vi "Multi1Darray.vi"() -> ()   [LabVIEW 2014]
uses:
  <vilib>/Analysis/baseanly.llb/Mean (DBL).vi
  <vilib>/Utility/file.llb/Read From Spreadsheet File (DBL).vi
  <vilib>/Analysis/NI_AALBase.lvlib
panel:
  out "Array":dbl[][](array[numeric])
  in  "Frame-rate correction":bool
  out "output array":path[][](array[path])=[[path "E:/MALDI Plots/02_14_24_data_18_spot_5_DHB_electrons_dwellandSample_5000_mcp_1850_phosphor_5500_range_2V_lens1_500_pump1.2probe0.2_4ps_3to48_backward_VelAcc_1_202402141810Cameracounts.dat"], [path "E:/MALDI Plots/02_14_24_data_14_spot_5_DHB_electrons_dwellandSample_5000_mcp_1850_phosphor_5500_range_2V_lens1_500_pump1.0probe0.2_4ps_3to48_backward_VelAcc_1_202402141718Cameracounts.dat"], [path "E:/MALDI Plots/02_14_24_data_12_spot_5_DHB_electrons_dwellandSample_5000_mcp_1850_phosphor_5500_range_2V_lens1_500_pump0.8probe0.2_4ps_3to48_backward_VelAcc_1_202402141651Cameracounts.dat"], [path "E:/MALDI Plots/02_14_24_data_10_spot_5_DHB_electrons_dwellandSample_5000_mcp_1850_phosphor_5500_range_2V_lens1_500_pump0.6probe0.2_4ps_3to48_backward_VelAcc_1_202402141629Cameracounts.dat"], [path "E:/MALDI Plots/02_14_24_data_2_spot_5_DHB_electrons_dwellandSample_5000_mcp_1850_phosphor_5500_range_2V_lens1_500_pump0.4probe0.2_4ps_3to48_backward_VelAcc_1_202402141222Cameracounts.dat"], [path "E:/MALDI Plots/02_13_24_data_6_spot_3_DHB_electrons_dwellandSample_5000_mcp_1850_phosphor_5500_range_2V_lens1_500_pump0.2probe0.2_1by1_4ps_3to48_backward_VelAcc_1_202402131406Cameracounts.dat"], [path ""], [path ""], [path ""]]
  in  "Stop Button":bool
  in  "start path":path=path "E:/MALDI Plots"
  in  "Tab Control":T1(tab)=enum."Combine Graph of 9 Plots"
  out "Waveform Graph 0":dbl[](graph)=[1.257, 1.248, 1.265, 1.215, 1.222, 1.21, 1.235, 1.2, 1.224, 1.247, 1.211, 1.189, 1.237, 1.208, 1.206, 1.211, 1.179, 1.203, 1.224, 1.217, 1.188, 1.224, 1.277, 1.3, 1.324, 1.333, 1.284, 1.238, 1.221, 1.215, 1.246, 1.229, 1.209, 1.228, 1.221, 1.194, 1.166, 1.215, 1.214, 1.184, 1.186, 1.221, 1.226, 1.218, 1.208, 1.187, 1.209, 1.166, 1.151, 1.201, 1.185, 1.164, 1.17, 1.155, 1.165, 1.181, 1.154, 1.211, 1.189, 1.174, 1.171, 1.169, 1.125, 1.173, 1.152, 1.2, 1.186, 1.178, 1.17, 1.166, 1.177, 1.171, 1.15, 1.15, 1.18]
  out "Waveform Graph 1":dbl[](graph)=[1.046, 1.067, 1.047, 1.058, 1.069, 1.074, 1.062, 1.069, 1.082, 1.057, 1.067, 1.081, 1.074, 1.099, 1.054, 1.069, 1.086, 1.073, 1.083, 1.068, 1.074, 1.106, 1.161, 1.261, 1.324, 1.33, 1.285, 1.249, 1.192, 1.194, 1.201, 1.196, 1.166, 1.155, 1.157, 1.152, 1.168, 1.131, 1.138, 1.109, 1.122, 1.112, 1.124, 1.086, 1.117, 1.102, 1.09, 1.096, 1.095, 1.098, 1.041, 1.053, 1.054, 1.061, 1.056, 1.057, 1.084, 1.074, 1.063, 1.061, 1.053, 1.052, 1.039, 1.042, 1.068, 1.058, 1.08, 1.082, 1.023, 1.028, 1.021, 1.008, 1.005, 1.05, 1.041]
  out "Waveform Graph 3":dbl[](graph)=[0.779, 0.736, 0.746, 0.749, 0.715, 0.75, 0.745, 0.769, 0.746, 0.78, 0.767, 0.765, 0.753, 0.755, 0.768, 0.746, 0.76, 0.76, 0.785, 0.784, 0.788, 0.772, 0.855, 0.958, 1.047, 1.097, 1.057, 1.034, 0.981, 0.982, 0.972, 0.963, 0.928, 0.922, 0.92, 0.915, 0.926, 0.887, 0.886, 0.869, 0.84, 0.84, 0.832, 0.822, 0.827, 0.816, 0.815, 0.831, 0.809, 0.816, 0.817, 0.805, 0.774, 0.765, 0.793, 0.83, 0.824, 0.802, 0.759, 0.776, 0.764, 0.743, 0.775, 0.762, 0.76, 0.77, 0.784, 0.761, 0.777, 0.763, 0.739, 0.746, 0.766, 0.746, 0.741]
  out "Waveform Graph 4":dbl[](graph)=[0.59, 0.604, 0.602, 0.59, 0.576, 0.579, 0.57, 0.581, 0.568, 0.579, 0.543, 0.58, 0.591, 0.577, 0.582, 0.563, 0.584, 0.591, 0.564, 0.571, 0.591, 0.625, 0.674, 0.786, 0.91, 0.973, 0.964, 0.935, 0.917, 0.899, 0.874, 0.844, 0.852, 0.817, 0.818, 0.8, 0.796, 0.769, 0.748, 0.732, 0.724, 0.717, 0.73, 0.699, 0.708, 0.685, 0.696, 0.701, 0.689, 0.651, 0.655, 0.663, 0.64, 0.653, 0.648, 0.665, 0.661, 0.616, 0.623, 0.634, 0.621, 0.633, 0.622, 0.617, 0.624, 0.614, 0.593, 0.606, 0.604, 0.573, 0.604, 0.586, 0.58, 0.558, 0.588]
  out "Waveform Graph 5":dbl[](graph)=[0.44, 0.48, 0.463, 0.455, 0.461, 0.469, 0.475, 0.477, 0.479, 0.482, 0.481, 0.477, 0.492, 0.492, 0.497, 0.495, 0.497, 0.511, 0.51, 0.503, 0.528, 0.535, 0.606, 0.734, 0.892, 0.981, 1.019, 0.964, 0.934, 0.887, 0.862, 0.851, 0.824, 0.85, 0.818, 0.791, 0.821, 0.761, 0.744, 0.739, 0.736, 0.722, 0.742, 0.681, 0.685, 0.668, 0.664, 0.678, 0.661, 0.643, 0.64, 0.644, 0.629, 0.601, 0.605, 0.594, 0.621, 0.612, 0.58, 0.546, 0.578, 0.569, 0.564, 0.58, 0.593, 0.569, 0.566, 0.559, 0.554, 0.555, 0.527, 0.518, 0.541, 0.541, 0.519]
  out "Waveform Graph 2":dbl[](graph)=[0.941, 0.927, 0.925, 0.947, 0.959, 0.926, 0.936, 0.927, 0.92, 0.909, 0.917, 0.929, 0.929, 0.912, 0.92, 0.92, 0.962, 0.937, 0.954, 0.958, 0.964, 0.964, 1.026, 1.13, 1.212, 1.247, 1.191, 1.156, 1.153, 1.094, 1.101, 1.071, 1.06, 1.046, 1.065, 1.035, 1.034, 1.025, 1.017, 1.015, 0.989, 1.009, 0.982, 0.977, 0.961, 0.994, 0.968, 0.948, 0.963, 0.964, 0.983, 0.924, 0.957, 0.947, 0.926, 0.94, 0.915, 0.942, 0.931, 0.916, 0.915, 0.922, 0.944, 0.907, 0.943, 0.922, 0.924, 0.916, 0.917, 0.919, 0.91, 0.911, 0.907, 0.9, 0.898]
  out "Waveform Graph 6":dbl[](graph)
  out "Waveform Graph 7":dbl[](graph)
  out "Waveform Graph 8":dbl[](graph)
  in  "Normalization method":u16(ring) items=["Raw Data", "Normalize to the peak", "Normalize to the baseline"]
  out "?":dbl[][](graph)=[[1.257, 1.248, 1.265, 1.215, 1.222, 1.21, 1.235, 1.2, 1.224, 1.247, 1.211, 1.189, 1.237, 1.208, 1.206, 1.211, 1.179, 1.203, 1.224, 1.217, 1.188, 1.224, 1.277, 1.3, 1.324, 1.333, 1.284, 1.238, 1.221, 1.215, 1.246, 1.229, 1.209, 1.228, 1.221, 1.194, 1.166, 1.215, 1.214, 1.184, 1.186, 1.221, 1.226, 1.218, 1.208, 1.187, 1.209, 1.166, 1.151, 1.201, 1.185, 1.164, 1.17, 1.155, 1.165, 1.181, 1.154, 1.211, 1.189, 1.174, 1.171, 1.169, 1.125, 1.173, 1.152, 1.2, 1.186, 1.178, 1.17, 1.166, 1.177, 1.171, 1.15, 1.15, 1.18], [1.046, 1.067, 1.047, 1.058, 1.069, 1.074, 1.062, 1.069, 1.082, 1.057, 1.067, 1.081, 1.074, 1.099, 1.054, 1.069, 1.086, 1.073, 1.083, 1.068, 1.074, 1.106, 1.161, 1.261, 1.324, 1.33, 1.285, 1.249, 1.192, 1.194, 1.201, 1.196, 1.166, 1.155, 1.157, 1.152, 1.168, 1.131, 1.138, 1.109, 1.122, 1.112, 1.124, 1.086, 1.117, 1.102, 1.09, 1.096, 1.095, 1.098, 1.041, 1.053, 1.054, 1.061, 1.056, 1.057, 1.084, 1.074, 1.063, 1.061, 1.053, 1.052, 1.039, 1.042, 1.068, 1.058, 1.08, 1.082, 1.023, 1.028, 1.021, 1.008, 1.005, 1.05, 1.041], [0.941, 0.927, 0.925, 0.947, 0.959, 0.926, 0.936, 0.927, 0.92, 0.909, 0.917, 0.929, 0.929, 0.912, 0.92, 0.92, 0.962, 0.937, 0.954, 0.958, 0.964, 0.964, 1.026, 1.13, 1.212, 1.247, 1.191, 1.156, 1.153, 1.094, 1.101, 1.071, 1.06, 1.046, 1.065, 1.035, 1.034, 1.025, 1.017, 1.015, 0.989, 1.009, 0.982, 0.977, 0.961, 0.994, 0.968, 0.948, 0.963, 0.964, 0.983, 0.924, 0.957, 0.947, 0.926, 0.94, 0.915, 0.942, 0.931, 0.916, 0.915, 0.922, 0.944, 0.907, 0.943, 0.922, 0.924, 0.916, 0.917, 0.919, 0.91, 0.911, 0.907, 0.9, 0.898], [0.779, 0.736, 0.746, 0.749, 0.715, 0.75, 0.745, 0.769, 0.746, 0.78, 0.767, 0.765, 0.753, 0.755, 0.768, 0.746, 0.76, 0.76, 0.785, 0.784, 0.788, 0.772, 0.855, 0.958, 1.047, 1.097, 1.057, 1.034, 0.981, 0.982, 0.972, 0.963, 0.928, 0.922, 0.92, 0.915, 0.926, 0.887, 0.886, 0.869, 0.84, 0.84, 0.832, 0.822, 0.827, 0.816, 0.815, 0.831, 0.809, 0.816, 0.817, 0.805, 0.774, 0.765, 0.793, 0.83, 0.824, 0.802, 0.759, 0.776, 0.764, 0.743, 0.775, 0.762, 0.76, 0.77, 0.784, 0.761, 0.777, 0.763, 0.739, 0.746, 0.766, 0.746, 0.741], [0.59, 0.604, 0.602, 0.59, 0.576, 0.579, 0.57, 0.581, 0.568, 0.579, 0.543, 0.58, 0.591, 0.577, 0.582, 0.563, 0.584, 0.591, 0.564, 0.571, 0.591, 0.625, 0.674, 0.786, 0.91, 0.973, 0.964, 0.935, 0.917, 0.899, 0.874, 0.844, 0.852, 0.817, 0.818, 0.8, 0.796, 0.769, 0.748, 0.732, 0.724, 0.717, 0.73, 0.699, 0.708, 0.685, 0.696, 0.701, 0.689, 0.651, 0.655, 0.663, 0.64, 0.653, 0.648, 0.665, 0.661, 0.616, 0.623, 0.634, 0.621, 0.633, 0.622, 0.617, 0.624, 0.614, 0.593, 0.606, 0.604, 0.573, 0.604, 0.586, 0.58, 0.558, 0.588], [0.44, 0.48, 0.463, 0.455, 0.461, 0.469, 0.475, 0.477, 0.479, 0.482, 0.481, 0.477, 0.492, 0.492, 0.497, 0.495, 0.497, 0.511, 0.51, 0.503, 0.528, 0.535, 0.606, 0.734, 0.892, 0.981, 1.019, 0.964, 0.934, 0.887, 0.862, 0.851, 0.824, 0.85, 0.818, 0.791, 0.821, 0.761, 0.744, 0.739, 0.736, 0.722, 0.742, 0.681, 0.685, 0.668, 0.664, 0.678, 0.661, 0.643, 0.64, 0.644, 0.629, 0.601, 0.605, 0.594, 0.621, 0.612, 0.58, 0.546, 0.578, 0.569, 0.564, 0.58, 0.593, 0.569, 0.566, 0.559, 0.554, 0.555, 0.527, 0.518, 0.541, 0.541, 0.519]]
  in  "Index":dbl
  in  "Length":dbl=150.0
  in  "Plot 1":u16(ring) items=["Plot 0", "Plot 1", "Plot 2", "Plot 3", "Plot 4", "Plot 5", "Plot 6", "Plot 7", "Plot 8"]
  in  "Feature On/Off":bool
  out "Combine graph 1":dbl[][](graph)=[[0.642, 0.631, 0.634, 0.632, 0.656, 0.666, 0.681, 0.659, 0.655, 0.66, 0.654, 0.682, 0.672, 0.695, 0.687, 0.674, 0.684, 0.688, 0.68, 0.693, 0.713, 0.731, 0.838, 1.072, 1.319, 1.442, 1.33, 1.313, 1.262, 1.224, 1.197, 1.191, 1.155, 1.137, 1.115, 1.122, 1.103, 1.1, 1.065, 1.058, 1.053, 1.007, 0.99, 0.942, 0.964, 0.979, 0.983, 0.953, 0.955, 0.977, 0.915, 0.931, 0.907, 0.912, 0.893, 0.91, 0.896, 0.927, 0.855, 0.878, 0.851, 0.854, 0.851, 0.839, 0.875, 0.828, 0.83, 0.804, 0.839, 0.834, 0.815, 0.791, 0.784, 0.784, 0.784], [0.634318732525629, 0.6625405405405406, 0.6517893755824791, 0.6168480894687792, 0.6585088536812675, 0.6611966449207829, 0.6625405405405406, 0.6571649580615098, 0.6544771668219944, 0.6719478098788444, 0.6706039142590866, 0.6732917054986021, 0.6638844361602982, 0.630287045666356, 0.6638844361602982, 0.6450698974836906, 0.6558210624417521, 0.6719478098788444, 0.6638844361602982, 0.6504454799627213, 0.6638844361602982, 0.6370065237651444, 0.6289431500465984, 0.7176402609506058, 0.936695246971109, 1.1624697110904008, 1.3559906803355077, 1.4057148182665424, 1.442, 1.3707735321528425, 1.394963653308481, 1.321049394221808, 1.358678471575023, 1.3237371854613234, 1.307610438024231, 1.278044734389562, 1.2740130475302889, 1.268637465051258, 1.2807325256290774, 1.186659832246039, 1.235040074557316, 1.2054743709226468, 1.1449990680335507, 1.153062441752097, 1.1369356943150046, 1.1221528424976701, 1.1033383038210625, 1.0898993476234857, 1.1019944082013047, 1.0952749301025164, 1.0858676607642126, 1.067053122087605, 1.0482385834109973, 1.0253923578751165, 0.9796999068033551, 0.9891071761416589, 1.0038900279589935, 0.9917949673811742, 0.9891071761416589, 0.9917949673811742, 0.9810438024231127, 0.9501342031686859, 0.9487903075489281, 0.9595414725069897, 0.9689487418452936, 0.9581975768872321, 0.9635731593662628, 0.9783560111835973, 0.9985144454799627, 0.9770121155638397, 0.9877632805219012, 0.9783560111835973, 0.9837315936626282, 0.9985144454799627, 1.0065778191985089]]
  in  "Offset":i32
  in  "Reverse":bool=TRUE
  in  "Select the plots to average":u16(ring)=2 items=["Plot 0", "Plot 1", "Plot 0 and Plot 1"]
  in  "Average criteria":i32=1
  in  "Plot 2":u16(ring) items=["Plot 0", "Plot 1", "Plot 2", "Plot 3", "Plot 4", "Plot 5", "Plot 6", "Plot 7", "Plot 8"]
  in  "Feature On/Off":bool
  out "Waveform Graph 10":dbl[][](graph)
  in  "Array 2":dbl[](array[numeric])
  in  "Length":dbl
  in  "Index":dbl
  out "best fit parameters":dbl[](array[numeric])
  out "Decay time constant from d":dbl=inf
  out "Decay time constant from b":dbl=inf
  out "XY Graph":cluster{dbl[], dbl[]}[](graph)
  in  "Step size (us)":dbl
  in  "Initial delay (us)":dbl
  # "Plot 0"
  # "Plot 1"
  # "Plot 2"
  # "Plot 3"
  # "Plot 4"
  # "Plot 5"
  # "Plot 6"
  # "Plot 7"
  # "Plot 8"
  # "a"
  # "b"
  # "c"
  # "d"
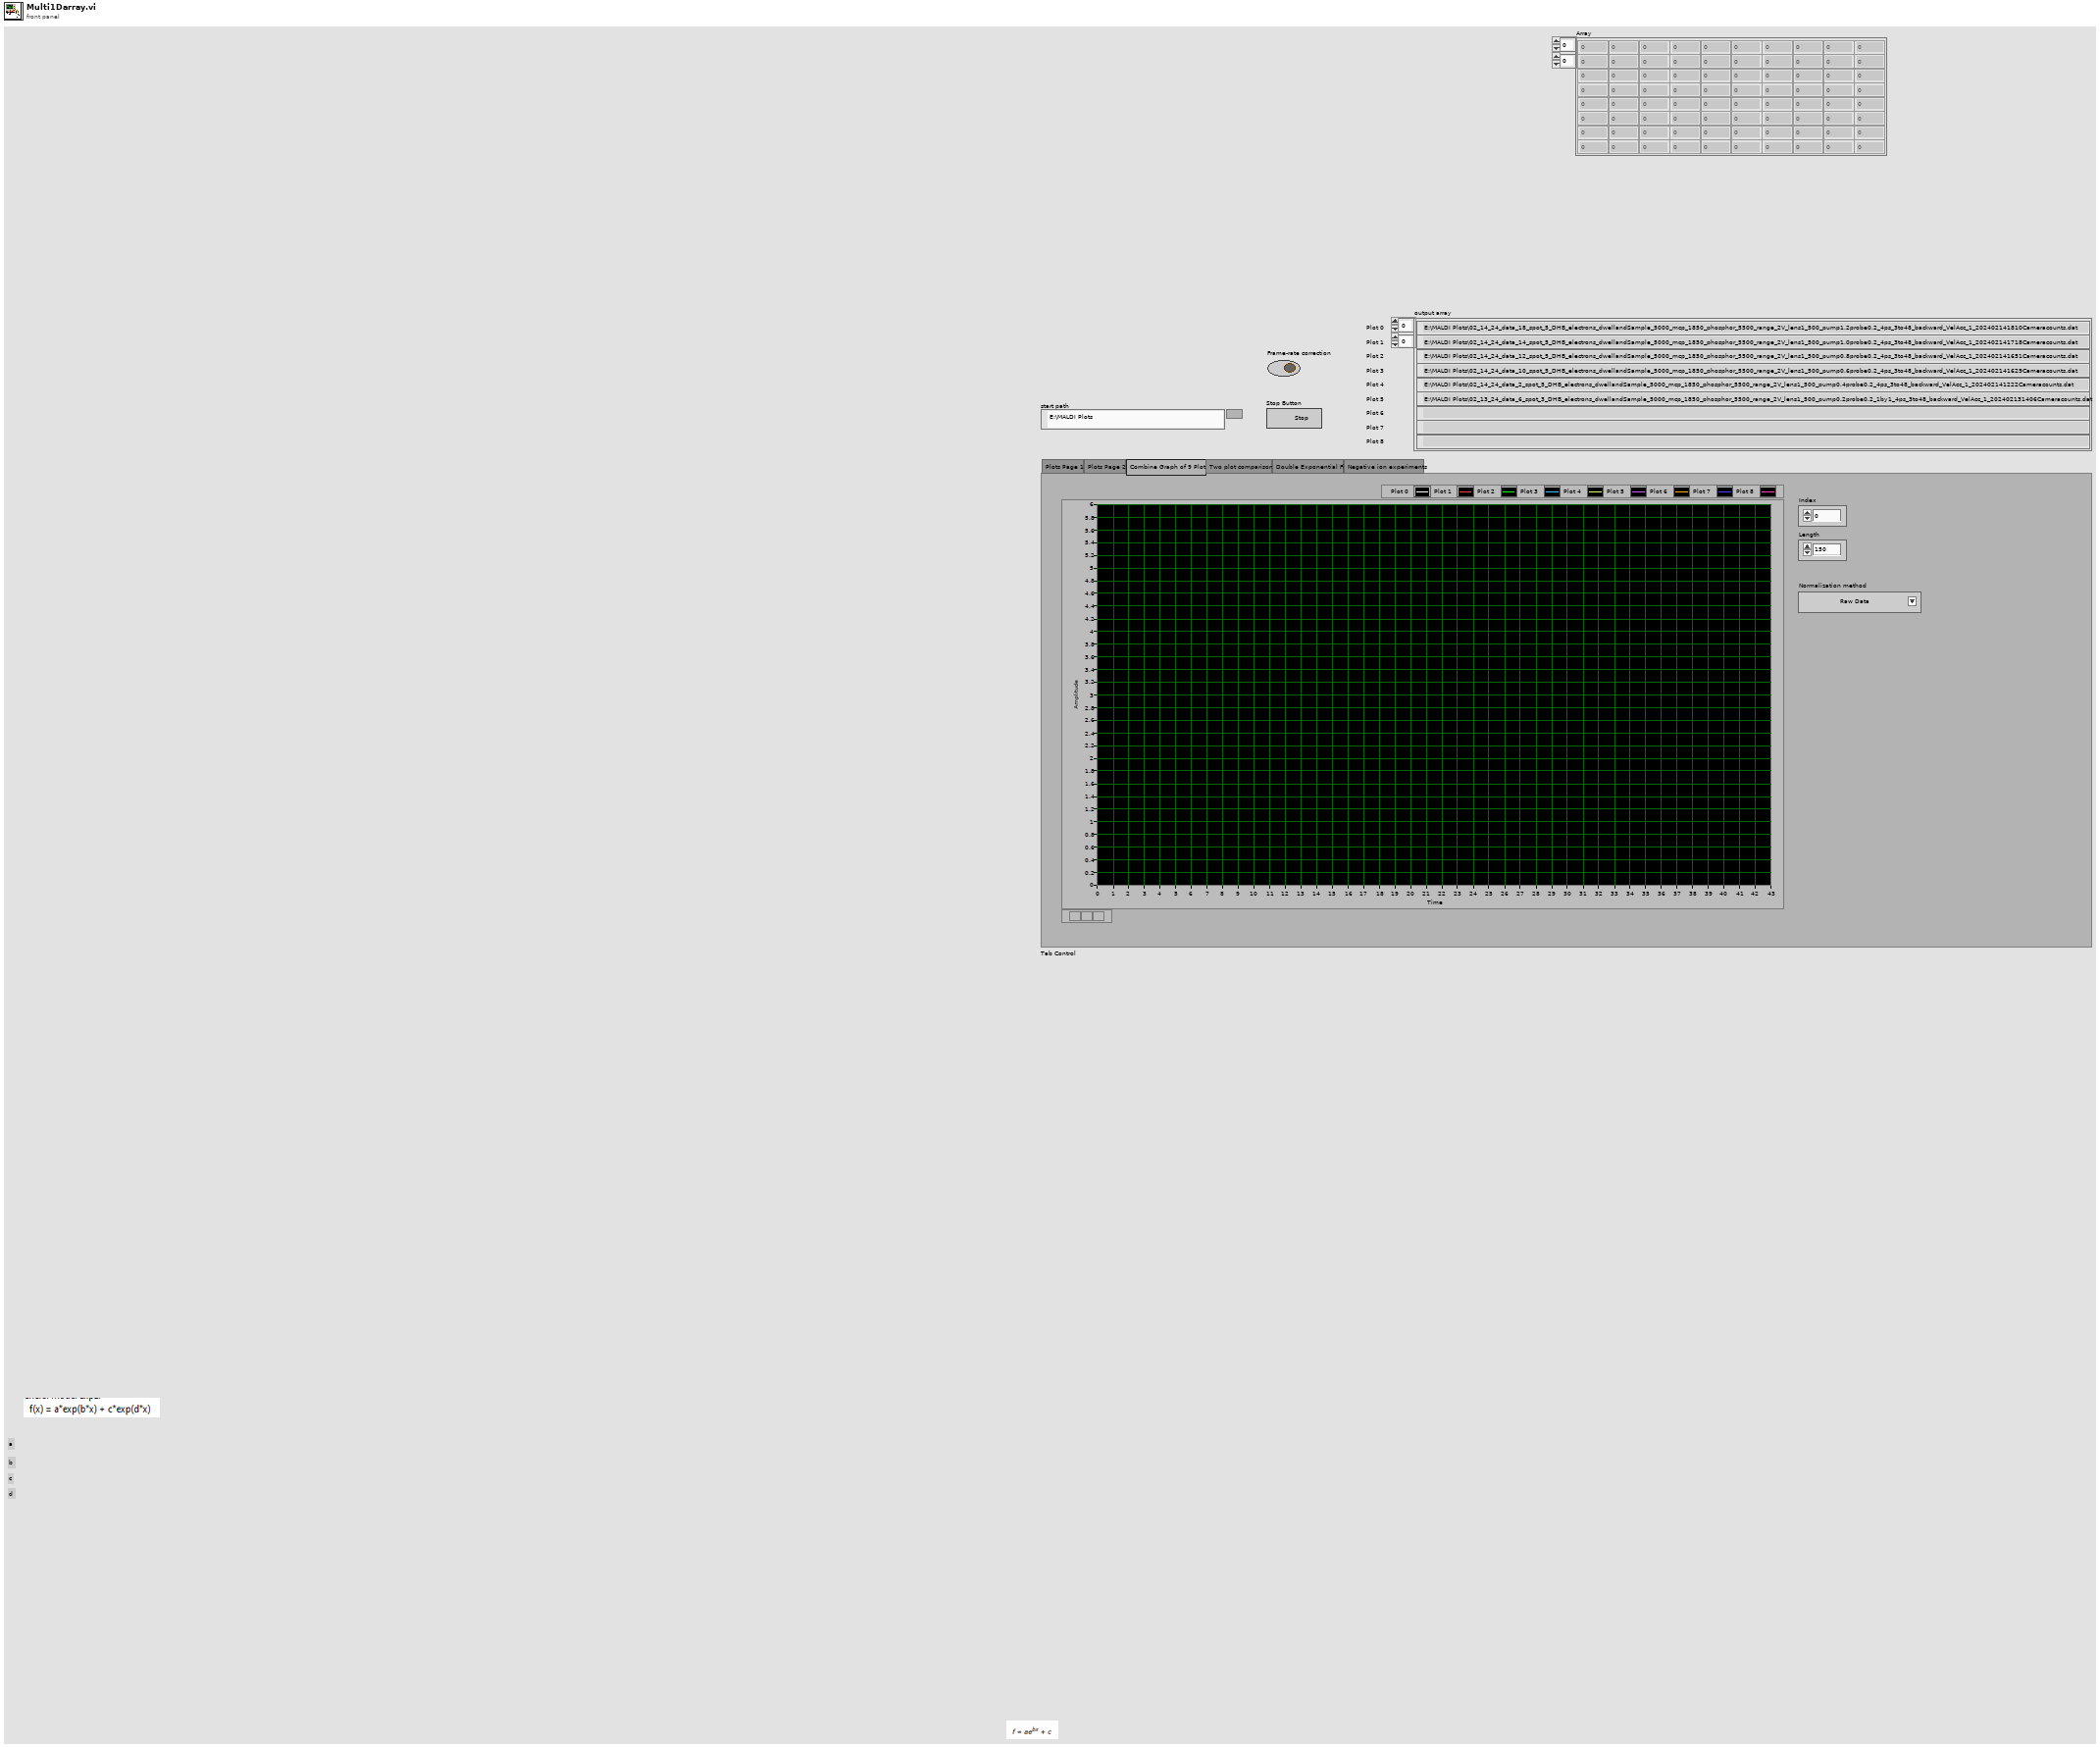
[diagram p1: front panel]
types:
  T1 = enum32{"Plots Page 1", "Plots Page 2", "Combine Graph of 9 Plots", "Two plot comparison", "Double Exponential Fit", "Negative ion experiments"}
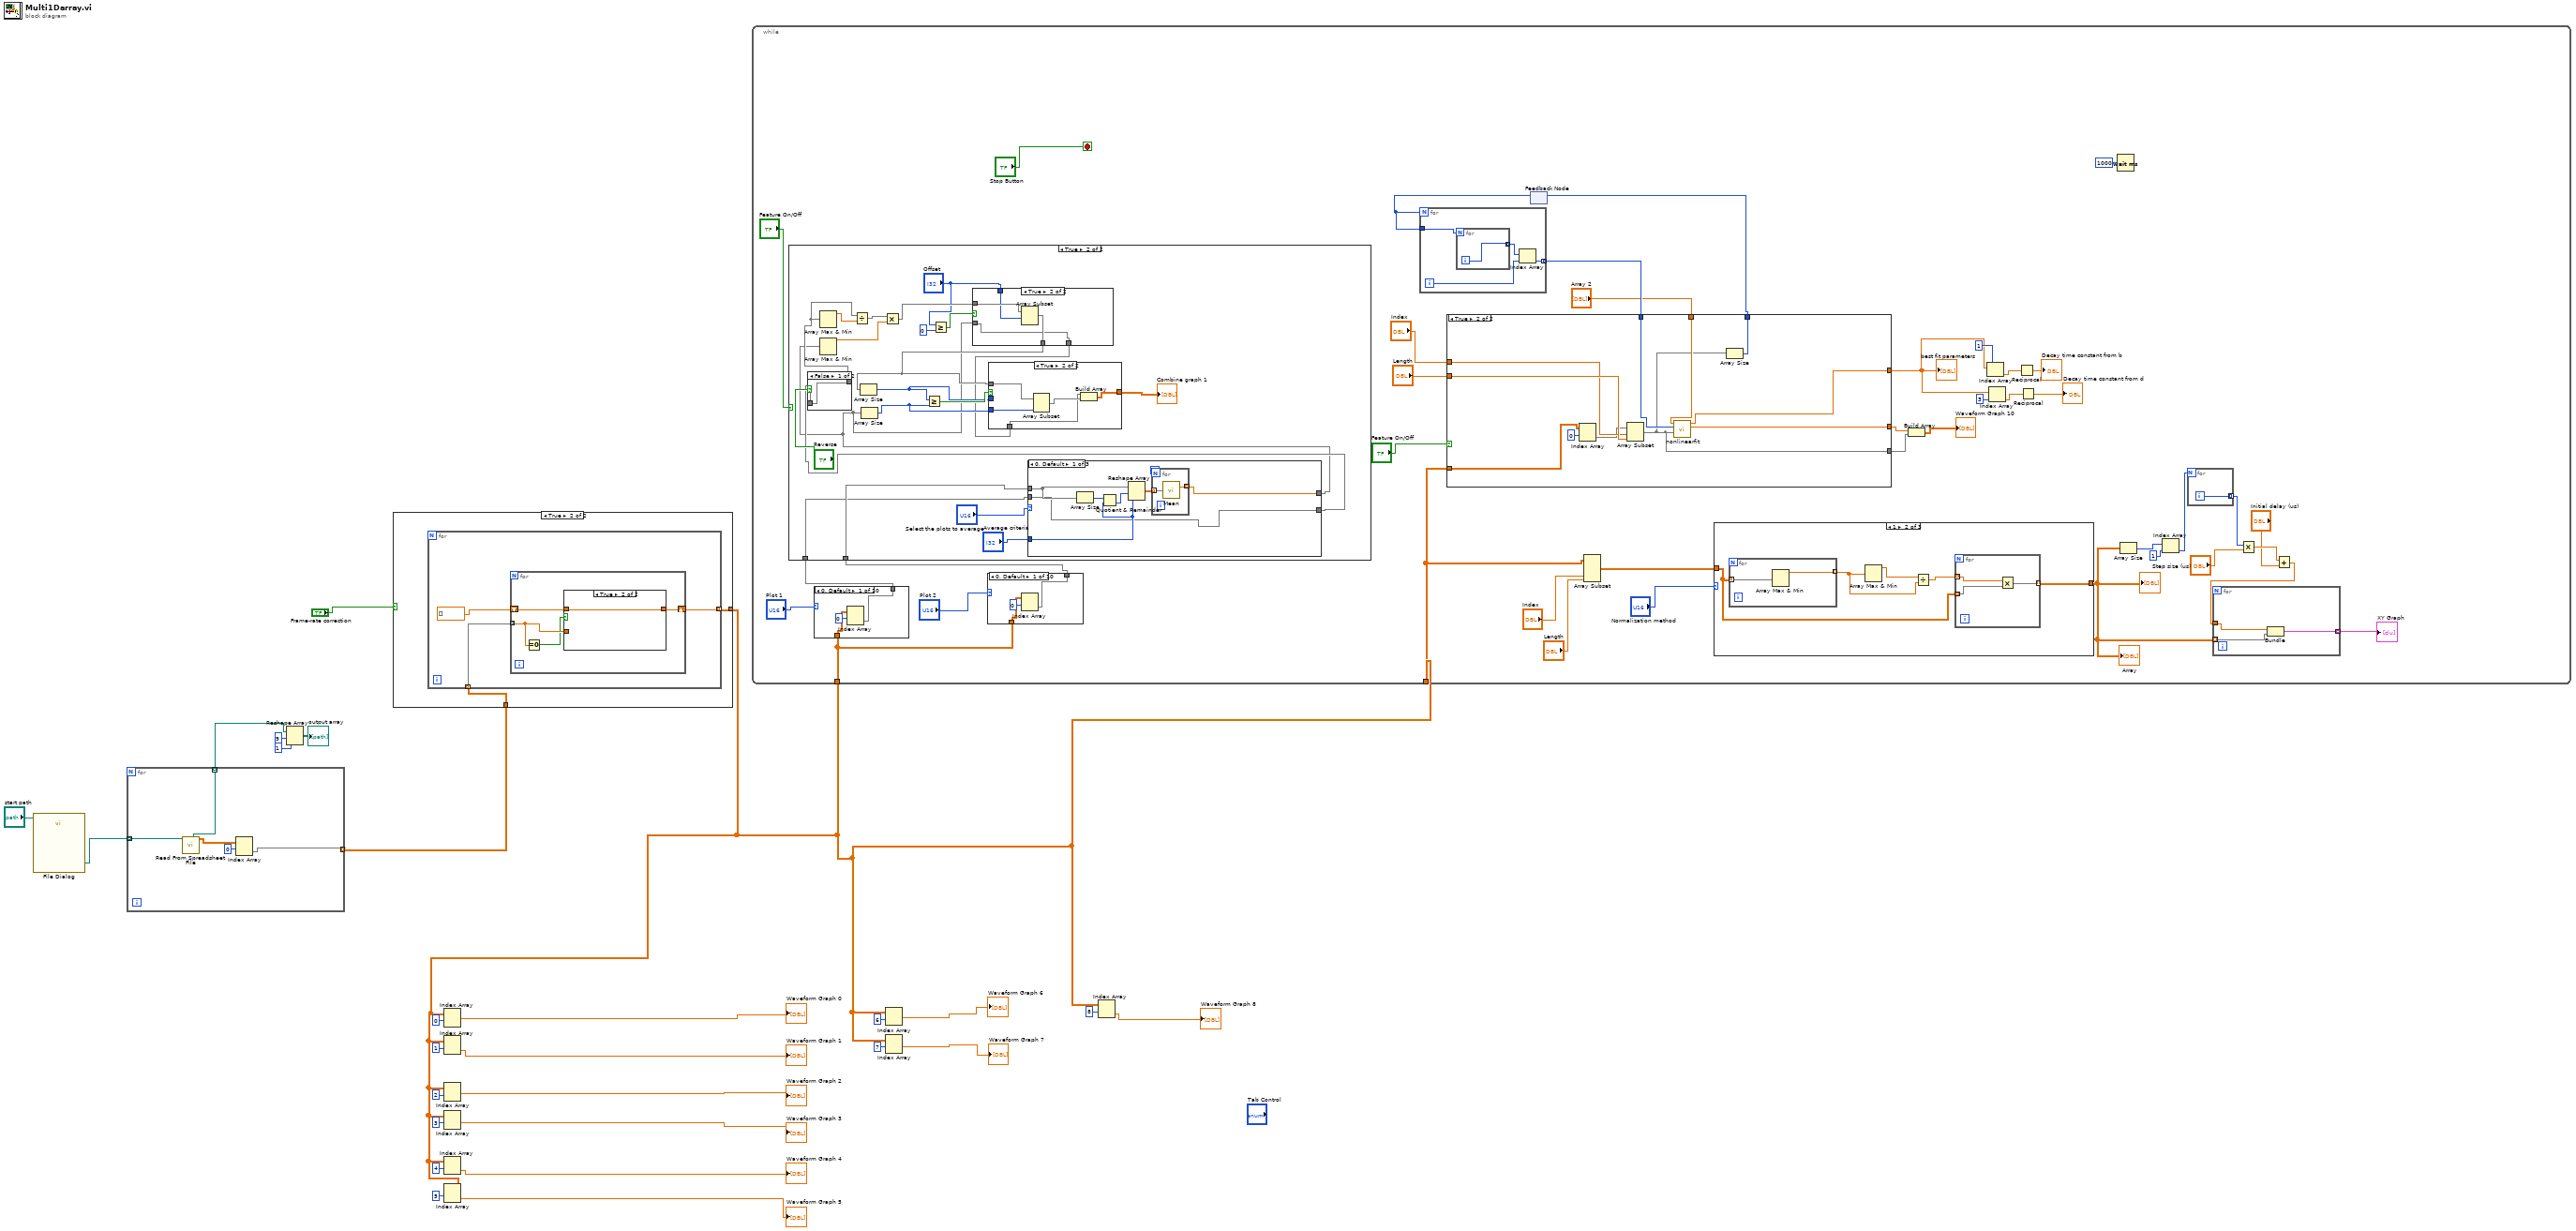
[diagram p0: block diagram]
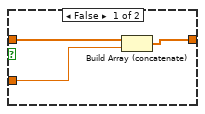
[diagram p3: hidden frame]
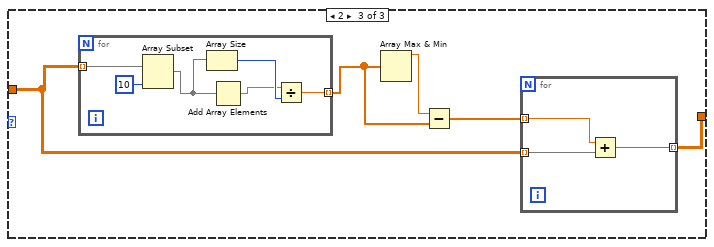
[diagram p5: hidden frame]
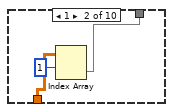
[diagram p6: hidden frame]
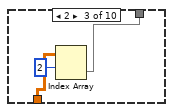
[diagram p7: hidden frame]
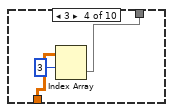
[diagram p8: hidden frame]
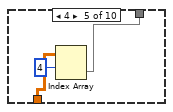
[diagram p9: hidden frame]
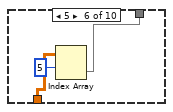
[diagram p10: hidden frame]
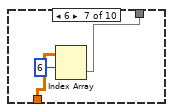
[diagram p11: hidden frame]
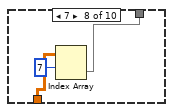
[diagram p12: hidden frame]
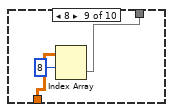
[diagram p13: hidden frame]
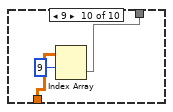
[diagram p14: hidden frame]
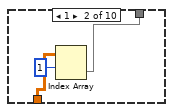
[diagram p15: hidden frame]
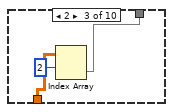
[diagram p16: hidden frame]
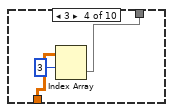
[diagram p17: hidden frame]
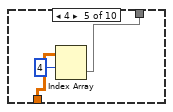
[diagram p18: hidden frame]
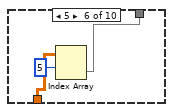
[diagram p19: hidden frame]
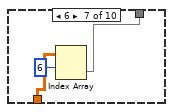
[diagram p20: hidden frame]
diagram:
  n1 = call "File Dialog"("start path"="start path") -> ("selected paths"=w26:path[])  [unwired: 11 in, 3 out]
  n2 = for {
    tunnel: w26 -> [w32] mode=indexing
    tunnel: [w29] -> w2 mode=indexing
    tunnel: [w28] -> w4 mode=indexing
    n3 = call-poly <vilib>:"Read From Spreadsheet File.vi"("file path (dialog if empty)"=w32) -> ("all rows"=w31:dbl[][], "new file path (Not A Path if cancelled)"=w28:path)  [unwired: 6 in, 3 out]
    n4 = Index Array(array=w31, index (row)=0) -> (element=w29:dbl[])  [unwired: 1 in]
  }
  n5 = Reshape Array(w4, 9 ("dimension size"), 1 ("dimension size")) -> (→"output array":path[][])
  n6 = case shown="True" "Frame-rate correction" {
    tunnel: w2 -> [w33 w35]
    tunnel: [w33 w34] -> w1
    frame False {
    }
    frame True {
      n7 = for {
        tunnel: w35 -> [w37] mode=indexing
        tunnel: [w36] -> w34 mode=indexing
        n8 = for {
          tunnel: w37 -> [w40] mode=indexing
          shift-right: [w41] -> w36
          shift-left: dbl[] [] -> [w42]
          n9 = Equal To 0?(x=w40) -> (x = 0?=w39:bool)
          n10 = case shown="True" w39 {
            tunnel: w40 -> [w45 _]
            tunnel: w42 -> [w44 w46]
            tunnel: [w43 w46] -> w41
            frame False {
              n11 = Build Array (concatenate)(w44, w45) -> (w43:dbl[])
            }
            frame True {
            }
          }
        }
      }
    }
  }
  n12 = Index Array(array=w1, index (row)=0) -> (element=→"Waveform Graph 0":dbl[])  [unwired: 1 in]
  n13 = Index Array(array=w1, index (row)=1) -> (element=→"Waveform Graph 1":dbl[])  [unwired: 1 in]
  n14 = Index Array(array=w1, index (row)=2) -> (element=→"Waveform Graph 2":dbl[])  [unwired: 1 in]
  n15 = Index Array(array=w1, index (row)=3) -> (element=→"Waveform Graph 3":dbl[])  [unwired: 1 in]
  n16 = Index Array(array=w1, index (row)=4) -> (element=→"Waveform Graph 4":dbl[])  [unwired: 1 in]
  n17 = Index Array(array=w1, index (row)=5) -> (element=→"Waveform Graph 5":dbl[])  [unwired: 1 in]
  n18 = while {
    tunnel: w1 -> [w60]
    tunnel: w1 -> [w78]
    stop <- "Stop Button" stop-if-true
    n19 = case shown="0, Default" "Plot 1" {
      tunnel: w78 -> [w148 w151 w154 w157 w160 w163 w166 w169 w172 w175]
      tunnel: [w147 w150 w153 w156 w159 w162 w165 w168 w171 w174] -> w79
      frame 0, Default {
        n20 = Index Array(array=w148, index (row)=0) -> (element=w147:dbl[])  [unwired: 1 in]
      }
      frame 1 {
        n21 = Index Array(array=w151, index (row)=1) -> (element=w150:dbl[])  [unwired: 1 in]
      }
      frame 2 {
        n22 = Index Array(array=w154, index (row)=2) -> (element=w153:dbl[])  [unwired: 1 in]
      }
      frame 3 {
        n23 = Index Array(array=w157, index (row)=3) -> (element=w156:dbl[])  [unwired: 1 in]
      }
      frame 4 {
        n24 = Index Array(array=w160, index (row)=4) -> (element=w159:dbl[])  [unwired: 1 in]
      }
      frame 5 {
        n25 = Index Array(array=w163, index (row)=5) -> (element=w162:dbl[])  [unwired: 1 in]
      }
      frame 6 {
        n26 = Index Array(array=w166, index (row)=6) -> (element=w165:dbl[])  [unwired: 1 in]
      }
      frame 7 {
        n27 = Index Array(array=w169, index (row)=7) -> (element=w168:dbl[])  [unwired: 1 in]
      }
      frame 8 {
        n28 = Index Array(array=w172, index (row)=8) -> (element=w171:dbl[])  [unwired: 1 in]
      }
      frame 9 {
        n29 = Index Array(array=w175, index (row)=9) -> (element=w174:dbl[])  [unwired: 1 in]
      }
    }
    n30 = case shown="0, Default" "Plot 2" {
      tunnel: w78 -> [w118 w121 w124 w127 w130 w133 w136 w139 w142 w145]
      tunnel: [w117 w120 w123 w126 w129 w132 w135 w138 w141 w144] -> w77
      frame 0, Default {
        n31 = Index Array(array=w118, index (row)=0) -> (element=w117:dbl[])  [unwired: 1 in]
      }
      frame 1 {
        n32 = Index Array(array=w121, index (row)=1) -> (element=w120:dbl[])  [unwired: 1 in]
      }
      frame 2 {
        n33 = Index Array(array=w124, index (row)=2) -> (element=w123:dbl[])  [unwired: 1 in]
      }
      frame 3 {
        n34 = Index Array(array=w127, index (row)=3) -> (element=w126:dbl[])  [unwired: 1 in]
      }
      frame 4 {
        n35 = Index Array(array=w130, index (row)=4) -> (element=w129:dbl[])  [unwired: 1 in]
      }
      frame 5 {
        n36 = Index Array(array=w133, index (row)=5) -> (element=w132:dbl[])  [unwired: 1 in]
      }
      frame 6 {
        n37 = Index Array(array=w136, index (row)=6) -> (element=w135:dbl[])  [unwired: 1 in]
      }
      frame 7 {
        n38 = Index Array(array=w139, index (row)=7) -> (element=w138:dbl[])  [unwired: 1 in]
      }
      frame 8 {
        n39 = Index Array(array=w142, index (row)=8) -> (element=w141:dbl[])  [unwired: 1 in]
      }
      frame 9 {
        n40 = Index Array(array=w145, index (row)=9) -> (element=w144:dbl[])  [unwired: 1 in]
      }
    }
    n41 = case shown="True" "Feature On/Off" {
      tunnel: w77 -> [_ w192]
      tunnel: w79 -> [_ w190]
      frame False {
      }
      frame True {
        n42 = Greater Or Equal?(x="Offset", y=0) -> (x >= y?=w194:bool)
        n43 = case shown="0, Default" "Select the plots to average" {
          tunnel: w192 -> [w210 w217 w227]
          tunnel: [w211 w217 w230] -> w188
          tunnel: "Average criteria" -> [w209 w221 w228]
          tunnel: w190 -> [w208 w220 w226]
          tunnel: [w208 w218 w229] -> w189
          frame 0, Default {
            n44 = Array Size(array=w210) -> (size(s)=w212:i32)
            n45 = Quotient & Remainder(x=w212, y=w209) -> (floor(x/y)=w213:i32)  [unwired: 1 out]
            n46 = Reshape Array(w210, w213, w209) -> (w214:dbl[][])
            n47 = for {
              tunnel: w214 -> [w216] mode=indexing
              tunnel: [w215] -> w211 mode=indexing
              n48 = call-poly <vilib>:"Mean.vi"("X"=w216) -> ("mean"=w215:dbl)  [unwired: 1 out]
            }
          }
          frame 1 {
            n49 = Array Size(array=w220) -> (size(s)=w222:i32)
            n50 = Quotient & Remainder(x=w222, y=w221) -> (floor(x/y)=w223:i32)  [unwired: 1 out]
            n51 = Reshape Array(w220, w223, w221) -> (w219:dbl[][])
            n52 = for {
              tunnel: w219 -> [w225] mode=indexing
              tunnel: [w224] -> w218 mode=indexing
              n53 = call-poly <vilib>:"Mean.vi"("X"=w225) -> ("mean"=w224:dbl)  [unwired: 1 out]
            }
          }
          frame 2 {
            n54 = Array Size(array=w227) -> (size(s)=w235:i32)
            n55 = Quotient & Remainder(x=w235, y=w228) -> (floor(x/y)=w236:i32)  [unwired: 1 out]
            n56 = Reshape Array(w227, w236, w228) -> (w234:dbl[][])
            n57 = for {
              tunnel: w234 -> [w240] mode=indexing
              tunnel: [w239] -> w230 mode=indexing
              n58 = call-poly <vilib>:"Mean.vi"("X"=w240) -> ("mean"=w239:dbl)  [unwired: 1 out]
            }
            n59 = Array Size(array=w226) -> (size(s)=w232:i32)
            n60 = Quotient & Remainder(x=w232, y=w228) -> (floor(x/y)=w233:i32)  [unwired: 1 out]
            n61 = Reshape Array(w226, w233, w228) -> (w231:dbl[][])
            n62 = for {
              tunnel: w231 -> [w238] mode=indexing
              tunnel: [w237] -> w229 mode=indexing
              n63 = call-poly <vilib>:"Mean.vi"("X"=w238) -> ("mean"=w237:dbl)  [unwired: 1 out]
            }
          }
        }
        n64 = case shown="False" "Reverse" {
          tunnel: w189 -> [w250 w252]
          tunnel: [w250 w251] -> w203
          frame False {
          }
          frame True {
            n65 = Reverse 1D Array(array=w252) -> (reversed array=w251:dbl[])
          }
        }
        n66 = Array Max & Min(array=w203) -> (max value=w202:dbl)  [unwired: 3 out]
        n67 = Array Max & Min(array=w188) -> (max value=w201:dbl)  [unwired: 3 out]
        n68 = Divide(x=w203, y=w202) -> (x/y=w204:dbl[])
        n69 = Array Size(array=w188) -> (size(s)=w206:i32)
        n70 = Multiply(x=w204, y=w201) -> (x*y=w199:dbl[])
        n71 = case shown="True" w194 {
          tunnel: w199 -> [w243 w249]
          tunnel: [w243 w248] -> w198
          tunnel: w188 -> [w245 w246]
          tunnel: [w244 w246] -> w197
          tunnel: "Offset" -> [w242 w247]
          frame False {
            n72 = Negate(x=w242) -> (-x=w241:i32)
            n73 = Array Subset(array=w245, index=w241) -> (w244:dbl[])  [unwired: 1 in]
          }
          frame True {
            n74 = Array Subset(array=w249, index=w247) -> (w248:dbl[])  [unwired: 1 in]
          }
        }
        n75 = Array Size(array=w198) -> (size(s)=w205:i32)
        n76 = Greater Or Equal?(x=w205, y=w206) -> (x >= y?=w207:bool)
        n77 = case shown="True" w207 {
          tunnel: w198 -> [w253 w262]
          tunnel: w206 -> [_ w261]
          tunnel: w205 -> [w257 _]
          tunnel: w197 -> [w256 w258]
          tunnel: [w255 w260] -> w187
          frame False {
            n78 = Array Subset(array=w256, length=w257) -> (w254:dbl[])  [unwired: 1 in]
            n79 = Build Array(w254, w253) -> (w255:dbl[][])
          }
          frame True {
            n80 = Array Subset(array=w262, length=w261) -> (w259:dbl[])  [unwired: 1 in]
            n81 = Build Array(w258, w259) -> (w260:dbl[][])
          }
        }
        "Combine graph 1" <- w187
      }
    }
    n82 = feedback #1() -> (w63:i32)  [unwired: 1 in]
    n83 = for {
      N: w63 -> [_]
      tunnel: [w264] -> w83 mode=indexing
      tunnel: w63 -> [w263]
      i -> [w266]
      n84 = for {
        N: w263 -> [_]
        tunnel: [w267] -> w265 mode=indexing
        i -> [w267]
      }
      n85 = Index Array(array=w265, index=w266) -> (element=w264:i32)
    }
    n86 = case shown="True" "Feature On/Off" {
      tunnel: w60 -> [_ w186]
      tunnel: "Length" -> [_ w185]
      tunnel: "Index" -> [_ w184]
      tunnel: w83 -> [_ w183]
      tunnel: "Array 2" -> [_ w182]
      tunnel: [_ w181] -> w75
      tunnel: [_ w180] -> w69
      tunnel: [_ w179] -> w74
      tunnel: [_ w178] -> w64
      frame False {
      }
      frame True {
        n87 = Index Array(array=w186, index (row)=0) -> (element=w176:dbl[])  [unwired: 1 in]
        n88 = Array Subset(array=w176, index=w184, length=w185) -> (w179:dbl[])
        n89 = call "nonlinearfit.vi"("Y Values"=w179, "X Values"=w183, "initial parameters"=w182) -> ("best nonlinear fit"=w181:dbl[], "best fit parameters"=w180:dbl[])  [unwired: 7 in]
        n90 = Array Size(array=w179) -> (size(s)=w178:i32)
      }
    }
    "best fit parameters" <- w69
    n91 = feedback-in #1(w64) -> ()
    n92 = Array Subset(array=w60, index (col)="Index", length (col)="Length") -> (w59:dbl[][])  [unwired: 2 in]
    n93 = case shown="1" "Normalization method" {
      tunnel: w59 -> [w91 w93 w102]
      tunnel: [w91 w92 w106] -> w54
      frame 0, Default {
      }
      frame 1 {
        n94 = for {
          tunnel: w93 -> [w97] mode=indexing
          tunnel: [w98] -> w94 mode=indexing
          n95 = Array Max & Min(array=w97) -> (max value=w98:dbl)  [unwired: 3 out]
        }
        n96 = Array Max & Min(array=w94) -> (max value=w96:dbl)  [unwired: 3 out]
        n97 = Divide(x=w96, y=w94) -> (x/y=w95:dbl[])
        n98 = for {
          tunnel: w93 -> [w101] mode=indexing
          tunnel: w95 -> [w100] mode=indexing
          tunnel: [w99] -> w92 mode=indexing
          n99 = Multiply(x=w100, y=w101) -> (x*y=w99:dbl[])
        }
      }
      frame 2 {
        n100 = for {
          tunnel: w102 -> [w112] mode=indexing
          tunnel: [w107] -> w104 mode=indexing
          n101 = Array Subset(array=w112, length=10) -> (w110:dbl[])  [unwired: 1 in]
          n102 = Array Size(array=w110) -> (size(s)=w109:i32)
          n103 = Add Array Elements(numeric array=w110) -> (sum=w108:dbl)
          n104 = Divide(x=w108, y=w109) -> (x/y=w107:dbl)
        }
        n105 = Array Max & Min(array=w104) -> (max value=w105:dbl)  [unwired: 3 out]
        n106 = Subtract(x=w105, y=w104) -> (x-y=w103:dbl[])
        n107 = for {
          tunnel: [w115] -> w106 mode=indexing
          tunnel: w103 -> [w114] mode=indexing
          tunnel: w102 -> [w113] mode=indexing
          n108 = Add(x=w114, y=w113) -> (x+y=w115:dbl[])
        }
      }
    }
    "?" <- w54
    "Array" <- w54
    n109 = Build Array(w75, w74) -> (→"Waveform Graph 10":dbl[][])
    n110 = Index Array(array=w69, index=1) -> (element=w70:dbl)
    n111 = Index Array(array=w69, index=3) -> (element=w67:dbl)
    n112 = Reciprocal(x=w70) -> (1/x=→"Decay time constant from b":dbl)
    n113 = Reciprocal(x=w67) -> (1/x=→"Decay time constant from d":dbl)
    n114 = Wait (ms)(milliseconds to wait=u32 1000) -> ()  [unwired: 1 out]
    n115 = Array Size(array=w54) -> (size(s)=w57:i32[])
    n116 = Index Array(array=w57, index=1) -> (element=w55:i32)
    n117 = for {
      N: w55 -> [_]
      tunnel: [w90] -> w52 mode=indexing
      i -> [w90]
    }
    n118 = Multiply(x=w52, y="Step size (us)") -> (x*y=w50:dbl[])
    n119 = Add(x=w50, y="Initial delay (us)") -> (x+y=w48:dbl[])
    n120 = for {
      tunnel: w54 -> [w88] mode=indexing
      tunnel: w48 -> [w89]
      tunnel: [w87] -> w53 mode=indexing
      n121 = Bundle(w89, w88) -> (w87:cluster{dbl[], dbl[]})  [unwired: 1 in]
    }
    "XY Graph" <- w53
  }
  n122 = Index Array(array=w1, index (row)=6) -> (element=→"Waveform Graph 6":dbl[])  [unwired: 1 in]
  n123 = Index Array(array=w1, index (row)=7) -> (element=→"Waveform Graph 7":dbl[])  [unwired: 1 in]
  n124 = Index Array(array=w1, index (row)=8) -> (element=→"Waveform Graph 8":dbl[])  [unwired: 1 in]
